vi "AgilentDCSource gpibtalkVoltage.vi"(2 "error in":errorcluster, 4 "Send":string) -> (0 "error out":errorcluster, 1 "read":string="\n")   [LabVIEW 2014]
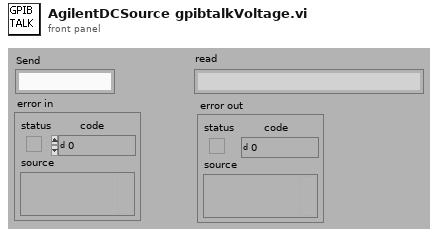
[diagram p1: front panel]
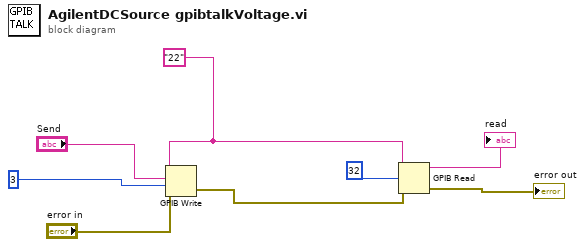
[diagram p0: block diagram]
diagram:
  w3 = "22"
  n1 = GPIB Write(0:w3, 1:"Send", 2:i16 3 ("mode (0)"), 3:"error in") -> (6:w8:errorcluster)  [unwired: 1 in, 1 out]
  n2 = GPIB Read(0:w3, 1:i16 32 ("mode (0)"), 3:w8) -> (5:→"read":string, 7:→"error out":errorcluster)  [unwired: 2 in, 1 out]
